vi "I2CWrite.vi"(6 "Timeout (10 s)":u8=10, 8 "error in (no error)":errorcluster, 9 "Number of Bytes to Write":u8, 10 "Data":u8[](array[numeric]), 11 "FPGA VI引用输入":refnum<k20>) -> (0 "error out":errorcluster, 3 "FPGA VI引用输出":refnum<k20>)   [LabVIEW 2015]
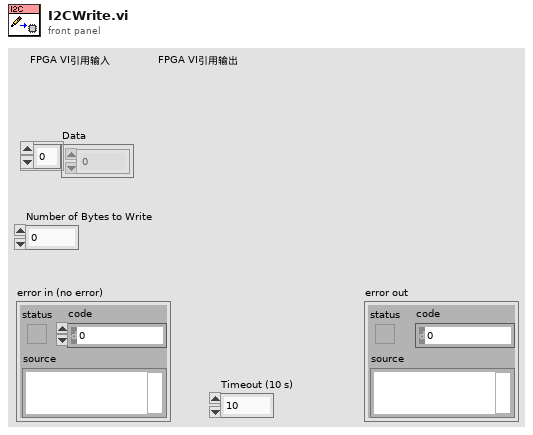
[diagram p1: front panel]
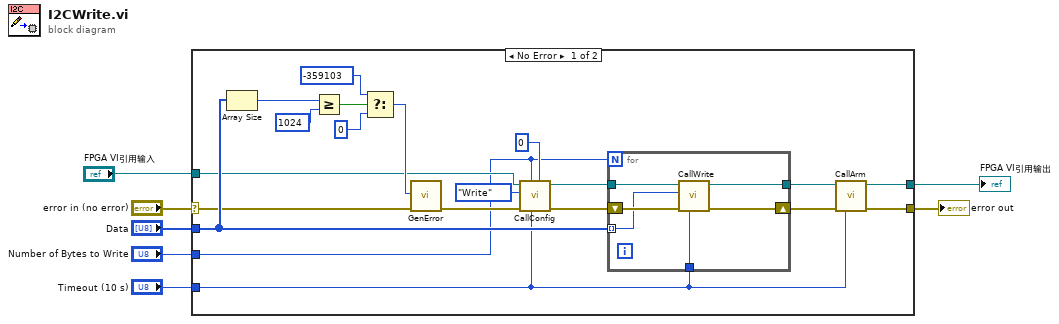
[diagram p0: block diagram]
diagram:
  n1 = case shown="No Error" "error in (no error)" {
    selector: "error in (no error)" -> [w21 w35]
    tunnel: "Data" -> [w27 _]
    tunnel: [w13 w35] -> w6
    tunnel: [w12 w34] -> w1
    tunnel: "Timeout (10 s)" -> [w8 _]
    tunnel: "FPGA VI引用输入" -> [w17 w34]
    tunnel: "Number of Bytes to Write" -> [w15 _]
    frame No Error {
      n2 = Array Size(array=w27) -> (size(s)=w22:i32)
      n3 = Greater Or Equal?(x=w22, y=1024) -> (x >= y?=w25:bool)
      n4 = Select(t=-359103 ("Code"), s=w25, f=0 ("Code")) -> (s? t:f=w20:i32)
      n5 = call "GenError.vi"("error in (no error)"=w21, "Code"=w20) -> ("error out"=w19:errorcluster)  [unwired: 9 in]
      n6 = call "CallConfig.vi"("Number of Bytes to Read"=u8 0, "Time out?"=w8, "Number of Bytes to Write"=w15, "error in (no error)"=w19, "Command"=enum16{"Write", "Read", "Write&Read"}."Write", "FPGA VI引用输入"=w17) -> ("error out"=w18:errorcluster, "FPGA VI引用输出"=w10:refnum<k20>)  [unwired: 4 in]
      n7 = for {
        N: w15 -> [_]
        tunnel: w27 -> [w31] mode=indexing
        shift-right: [w32] -> w14
        shift-left: w18 -> [w33]
        tunnel: w8 -> [w30]
        tunnel: [w29] -> w11
        tunnel: w10 -> [w28]
        n8 = call "CallWrite.vi"("Time out?"=w30, "error in (no error)"=w33, "Data"=w31, "FPGA VI引用输入"=w28) -> ("error out"=w32:errorcluster, "FPGA VI引用输出"=w29:refnum<k20>)  [unwired: 6 in]
      }
      n9 = call "CallArm.vi"("Time out?"=w8, "error in (no error)"=w14, "FPGA VI引用输入"=w11) -> ("error out"=w13:errorcluster, "FPGA VI引用输出"=w12:refnum<k20>)  [unwired: 7 in]
    }
    frame Error {
    }
  }
  "error out" <- w6
  "FPGA VI引用输出" <- w1
